vi "LINX - Blink (Simple).vi"() -> ()   [LabVIEW 2020]
uses:
  <vilib>/addons/Biomedical/Controls/Biosignal/Biosignal Spectrum/Biosignal Spectrum.xctl
  <vilib>/addons/Biomedical/Biosignal Measurements/ECG/subVIs/ECG features.ctl
  <vilib>/Analysis/3filter.llb/Filter Passband Type.ctl
  <vilib>/addons/Biomedical/Biosignal Measurements/ECG/HRV analysis/subVIs/bmt_HRV FFT Settings.ctl
  <vilib>/addons/Biomedical/Biosignal Measurements/ECG/HRV analysis/subVIs/bmt_HRV Frequency Bands.ctl
  <vilib>/addons/Biomedical/Biosignal Measurements/ECG/HRV analysis/subVIs/bmt_HRV AR Settings.ctl
  <vilib>/MakerHub/LINX/Public/Peripherals/Analog/Analog Read 1 Chan.vi
  <vilib>/MakerHub/LINX/Public/Peripherals/Analog/Analog Read N Chans.vi
  <vilib>/MakerHub/LINX/Private/Local IO/LinxAnalogRead.vi
  <vilib>/MakerHub/LINX/Public/Utilities/Check Channel.vi
  <vilib>/MakerHub/LINX/Public/Utilities/Open Serial.vi
  <vilib>/MakerHub/LINX/Private/Utilties/Generate Error.vi
  <vilib>/addons/Biomedical/Biosignal Measurements/ECG/ECG Feature Extractor (Array All).vi
  <vilib>/addons/Wavelet Analysis/application.llb/WA Detrend (Array).vi
  <vilib>/addons/Biomedical/Biosignal Measurements/ECG/HRV analysis/HRV FFT Spectrum (Array Unevenly Sampled RR).vi
  <vilib>/addons/Biomedical/Controls/Biosignal/HRV Spectrum Helper (FFT).vi
  <vilib>/addons/Biomedical/Biosignal Measurements/ECG/HRV analysis/HRV AR Spectrum (Array Unevenly Sampled RR).vi
  <vilib>/addons/Biomedical/Controls/Biosignal/HRV Spectrum Helper (AR).vi
  <vilib>/addons/Biomedical/Biosignal Measurements/ECG/HRV analysis/HRV STFT Spectrogram (Array Unevenly Sampled RR).vi
  <vilib>/addons/Time Frequency Analysis/_control.llb/TFA Configure Spectrogram Indicator (Predefined Color Table).vi
  <vilib>/MakerHub/LINX/LMH-LINX.lvlib
  <vilib>/addons/Biomedical/NI_BMTK_Measurements.lvlib
  <vilib>/ptbypt/NI_PtbyPt.lvlib
  <vilib>/Analysis/NI_AALBase.lvlib
  <vilib>/addons/Biomedical/NI_BMTK_Controls.lvlib
  <vilib>/addons/_Advanced Signal Processing/NI_AdvSigProcTFA.lvlib
  <vilib>/addons/_Advanced Signal Processing/NI_AdvSigProcWA.lvlib
panel:
  in  "Tab Control":T1(tab)
  out "NN50":i32
  out "pNN50":dbl format="%#.3g"
  out "RMSSD":dbl format="%#.3g ms"
  out "HR std":dbl format="%#.1g bpm"
  out "HR mean":dbl format="%#.1g bpm"
  out "RR std":dbl format="%#.3g s"
  out "RR mean":dbl format="%#.3g s"
  out "Count":i32
  out "RR interval histogram":T2(graph)
  out "RR triangular index":dbl format="%#_3g"
  out "TINN":dbl format="%#_3g ms"
  out "Poincare plot":cluster{"first row":dbl[], dbl[]}[](graph)
  out "SD1":dbl format="%0.2f ms"
  out "SD2":dbl format="%0.2f ms"
  out "FFT Spectrum":cluster{"f0":dbl, "df":dbl, "S(f)":dbl[]}(xcontrol)
  out "VLF Power (FFT)":dbl format="%#_2f ms^2"
  out "LF Power (FFT)":dbl format="%#_2f ms^2"
  out "HF Power (FFT)":dbl format="%#_2f ms^2"
  out "VLF [%] (FFT)":dbl format="%#_2f %"
  out "LF [%] (FFT)":dbl format="%#_2f %"
  out "HF [%] (FFT)":dbl format="%#_2f %"
  out "LF norm (FFT)":dbl format="%#_3f n.u."
  out "HF norm (FFT)":dbl format="%#_3f n.u."
  out "LF/HF (FFT)":dbl format="%#_2f"
  out "AR Spectrum":cluster{"f0":dbl, "df":dbl, "S(f)":dbl[]}(xcontrol)
  out "LF/HF (AR)":dbl format="%#_2f"
  out "HF norm (AR)":dbl format="%#_3f n.u."
  out "LF norm (AR)":dbl format="%#_3f n.u."
  out "HF [%] (AR)":dbl format="%#_2f %"
  out "LF [%] (AR)":dbl format="%#_2f %"
  out "VLF [%] (AR)":dbl format="%#_2f %"
  out "HF Power (AR)":dbl format="%#_2f ms^2"
  out "LF Power (AR)":dbl format="%#_2f ms^2"
  out "VLF Power (AR)":dbl format="%#_2f ms^2"
  out "Spectrogram":dbl[][](graph)
  out "ECG features array":T3[](array[typedef])
  out "RR interval":dbl
  out "final ECG ( without powerline noise and baseline wandering)":dbl[](graph)
  out "Statistics":T4 {"HR mean" format="%#_6f"}
  in  "Analog Input Channel":u8=13
  in  "Analyze Button":bool
  out "Loop Rate (Hz)":u32
  out "ECG without baseline wandering":dbl[](graph)
  out "original ECG":dbl[](graph)
  out "Instant Heart Rate":i32
  in  "Serial Port":refnum<visa-resource-name>
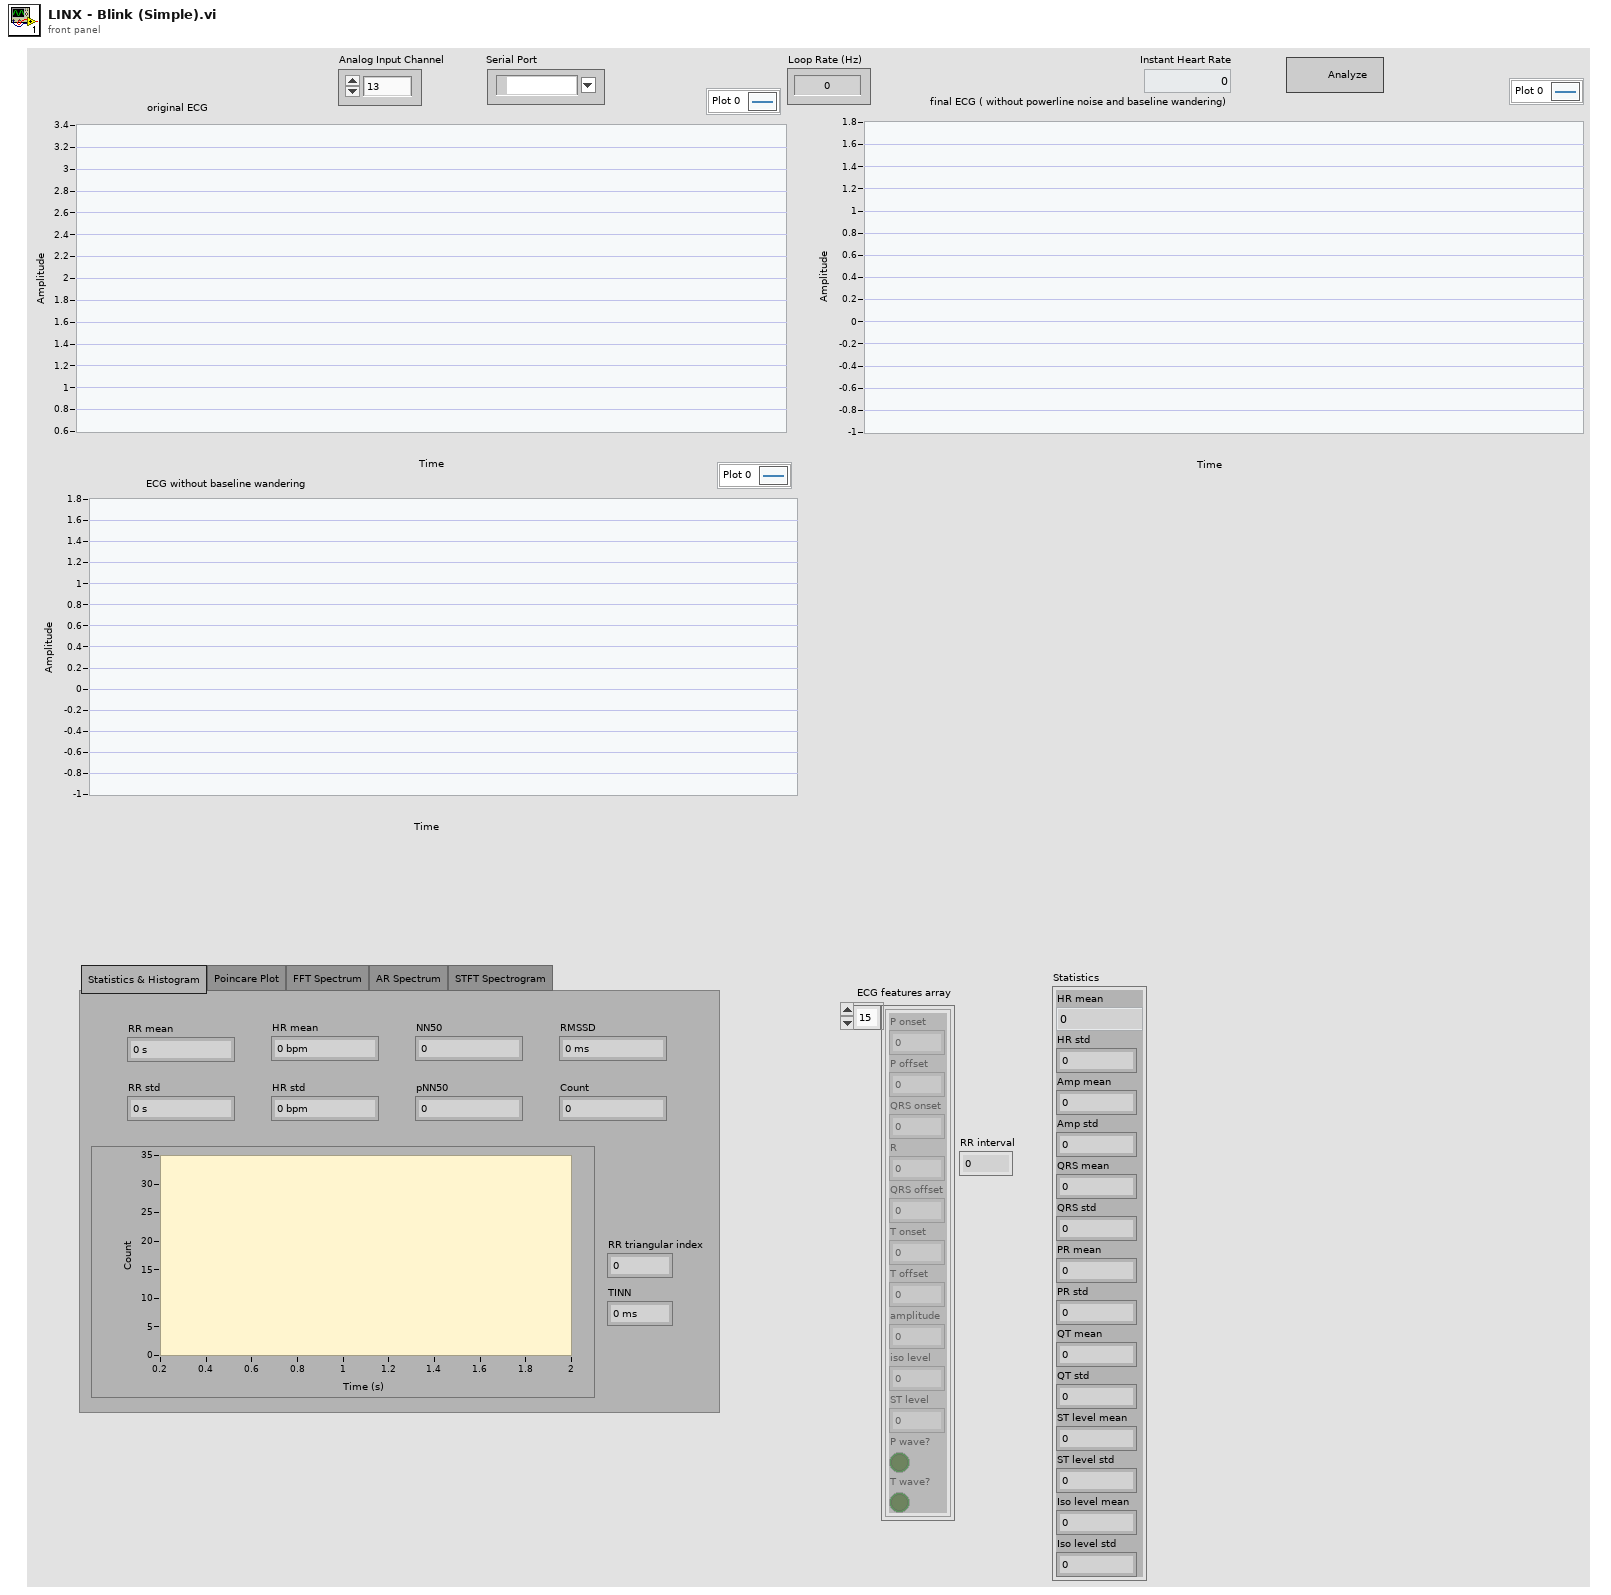
[diagram p1: front panel]
types:
  T1 = enum32{"Statistics & Histogram", "Poincare Plot", "FFT Spectrum", "AR Spectrum", "STFT Spectrogram"}
  T2 = cluster{"X Values":dbl[], "Histogram: h(x)":i32[]}
  T3 = typedef "NI_BMTK_Measurements.lvlib/ECG features.ctl" = cluster{"P onset":dbl, "P offset":dbl, "QRS onset":dbl, "R":dbl, "QRS offset":dbl, "T onset":dbl, "T offset":dbl, "amplitude":dbl, "iso level":dbl, "ST level":dbl, "P wave?":bool, "T wave?":bool}
  T4 = cluster{"HR mean":dbl, "HR std":dbl, "Amp mean":dbl, "Amp std":dbl, "QRS mean":dbl, "QRS std":dbl, "PR mean":dbl, "PR std":dbl, "QT mean":dbl, "QT std":dbl, "ST level mean":dbl, "ST level std":dbl, "Iso level mean":dbl, "Iso level std":dbl}
  T5 = typedef "NI_AALBase.lvlib/Filter Passband Type.ctl" = enum32{"Lowpass", "Highpass", "Bandpass", "Bandstop"}
  T6 = typedef "LMH-LINX.lvlib/LINX Ref.ctl" = cluster{"IO":T7, "Interface":T8, "LINX Device Config":T9}
  T7 = typedef "LMH-LINX.lvlib/Platform.ctl" = enum16{"Remote", "Local"}
  T8 = typedef "LMH-LINX.lvlib/Interface.ctl" = enum16{"Serial", "TCP"}
  T9 = typedef "LMH-LINX.lvlib/Device.lvlib/LINX Device Config.ctl" = cluster{"Interface":T8, "COM Port":refnum<visa-resource-name>, "TCP Configuration":T10, "Device Family":u8, "Device ID":u8, "Device Name":string, "TCP Ref":refnum<k5>, "Channels":T11}
  T10 = typedef "LMH-LINX.lvlib/Device.lvlib/TCP Config.ctl" = cluster{"IP Address":string, "Port":u16}
  T11 = typedef "LMH-LINX.lvlib/Channels.ctl" = cluster{"DI":u8[], "DO":u8[], "AI":u8[], "AO":u8[], "PWM":u8[], "QE":u8[], "UART":u8[], "I2C 2":u8[], "SPI":u8[], "CAN":u8[], "Servo":u8[], "AI Ref (V)":dbl, "AI Resolution (Bits)":u8, "AO Ref (V)":dbl, "AO Resolution (Bits)":u8}
  T12 = typedef "NI_BMTK_Measurements.lvlib/hrv statistics measures.ctl" = cluster{"NN50":i32, "pNN50":dbl, "RMSSD":dbl, "HR std":dbl, "HR mean":dbl, "RR std ":dbl, "RR mean":dbl}
  T13 = typedef "NI_BMTK_Measurements.lvlib/bmt_HRV FFT Settings.ctl" = cluster{"window settings":cluster{"window":u16, "length":i32, "overlap [%]":dbl}, "frequency bands":T14, "dB on? (F)":bool, "frequency bins":i32}
  T14 = typedef "NI_BMTK_Measurements.lvlib/bmt_HRV Frequency Bands.ctl" = cluster{"VLF high":dbl, "VLF low":dbl, "LF high":dbl, "LF low":dbl, "HF high":dbl, "HF low":dbl}
  T15 = typedef "NI_BMTK_Measurements.lvlib/bmt_Spectrum Meatures.ctl" = cluster{"VLF peak frequency":dbl, "VLF peak amplitude ":dbl, "LF peak frequency ":dbl, "LF peak amplitude ":dbl, "HF peak frequency":dbl, "HF peak amplitude":dbl, "VLF power":dbl, "LF power":dbl, "HF power":dbl, "LF norm":dbl, "HF norm":dbl, "LF/HF":dbl, "VLF [%]":dbl, "LF [%]":dbl, "HF [%]":dbl}
  T16 = typedef "NI_BMTK_Measurements.lvlib/bmt_HRV AR Settings.ctl" = cluster{"frequency bands":T14, "dB on? (F)":bool, "method":u16, "order":i32, "frequency bins":i32}
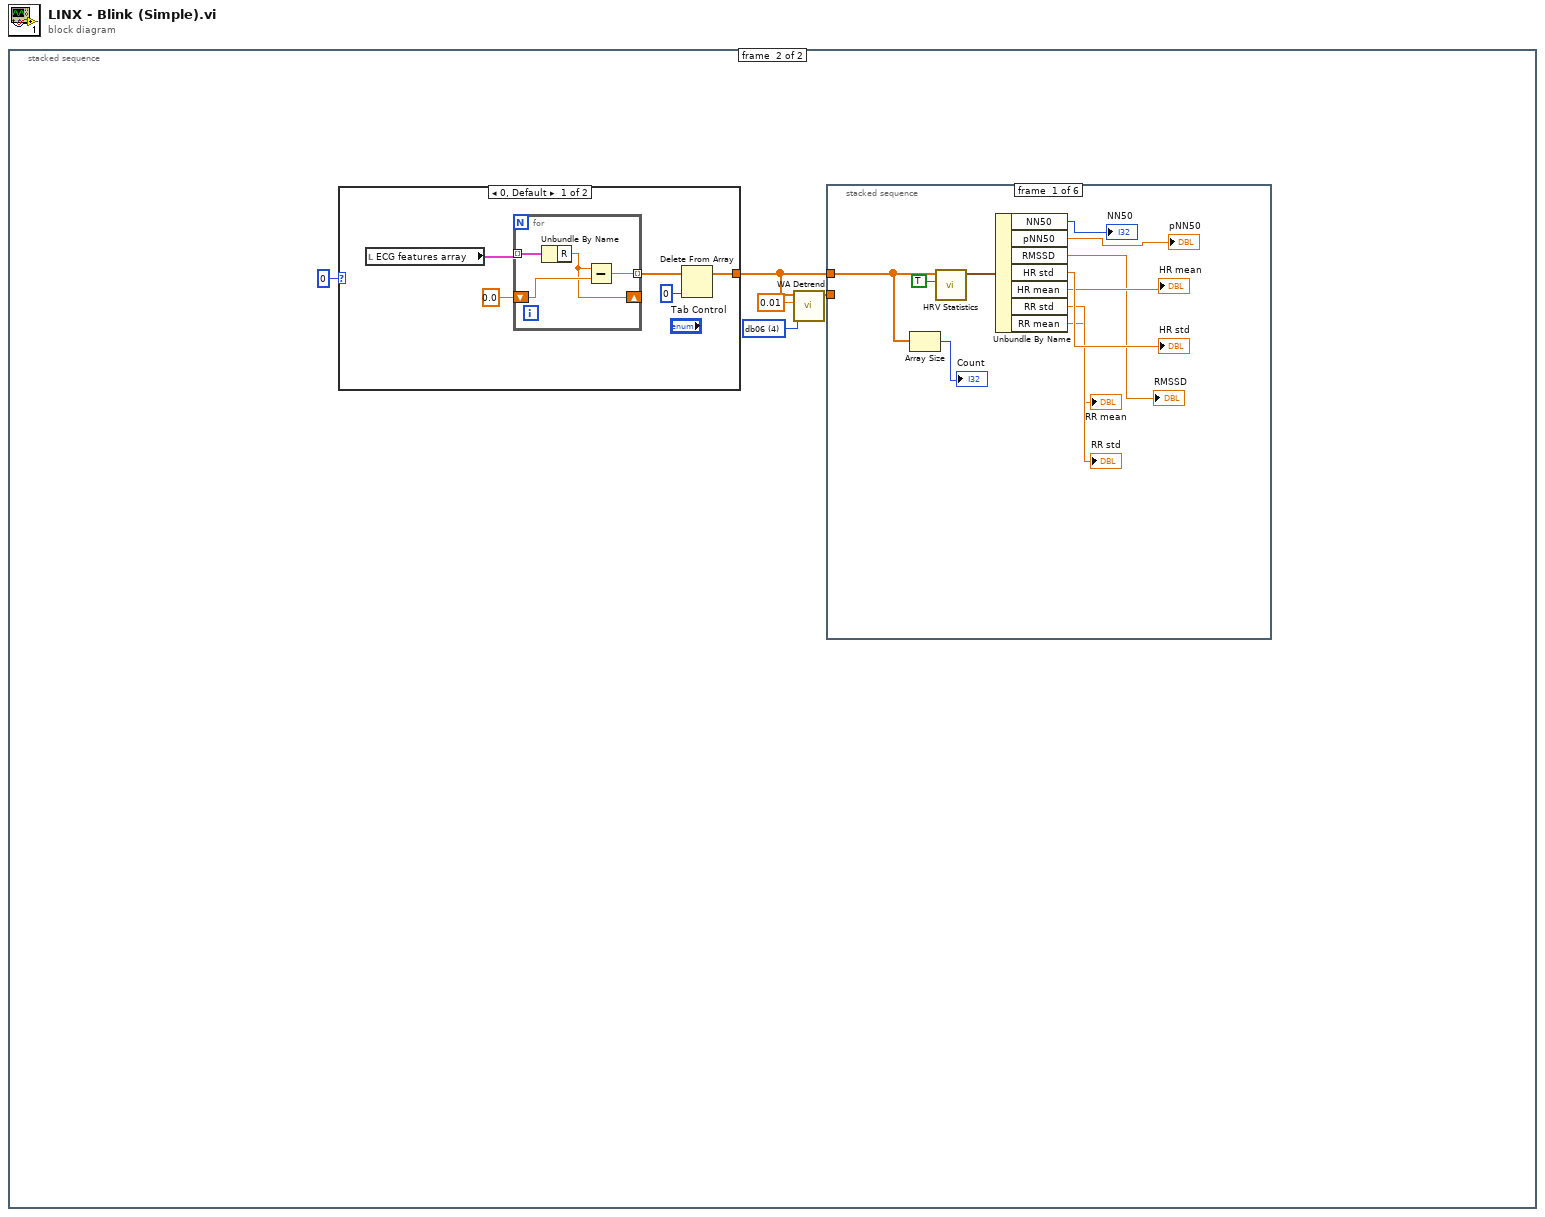
[diagram p0: block diagram]
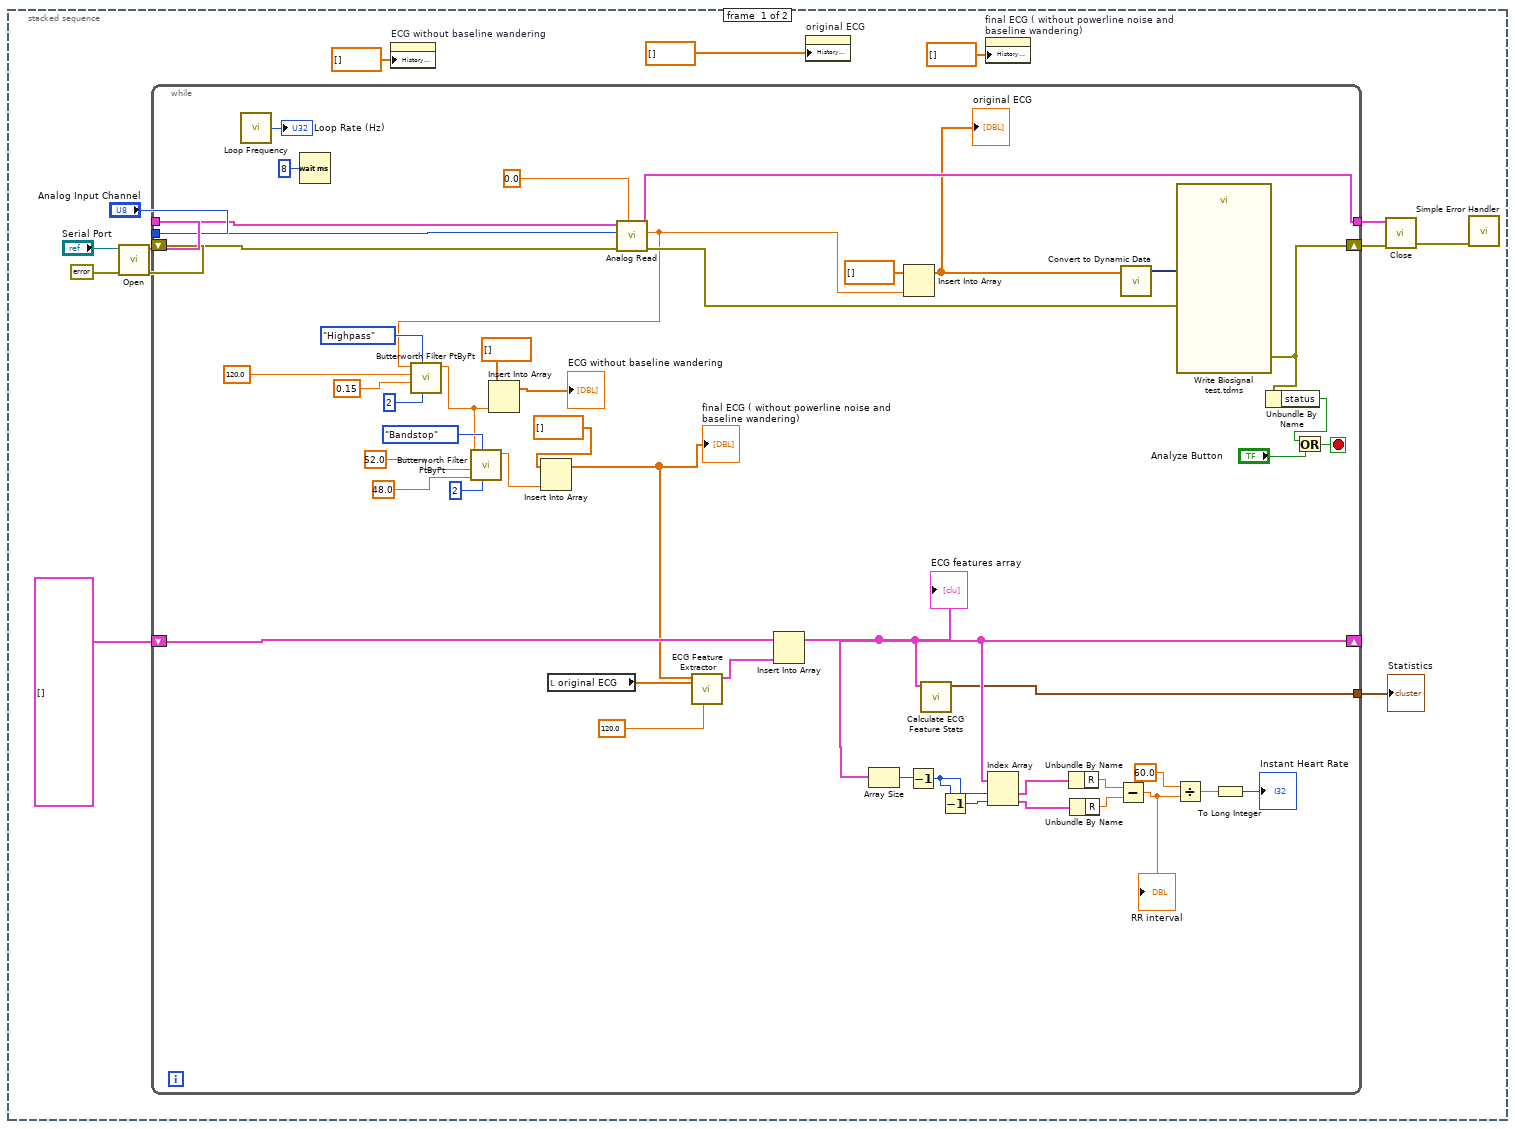
[diagram p2: hidden frame]
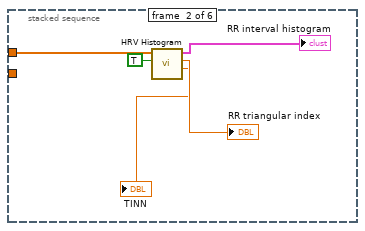
[diagram p3: hidden frame]
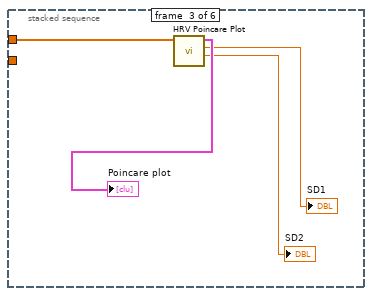
[diagram p4: hidden frame]
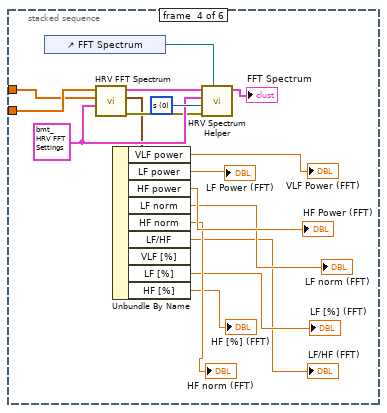
[diagram p5: hidden frame]
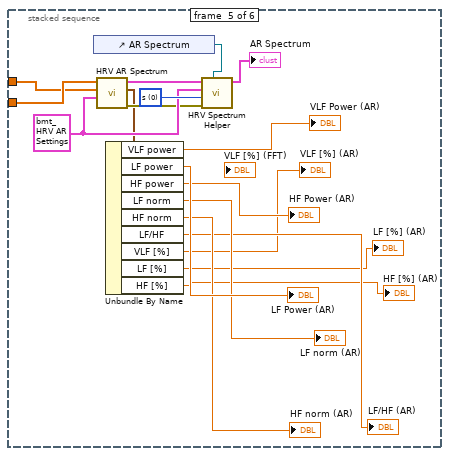
[diagram p6: hidden frame]
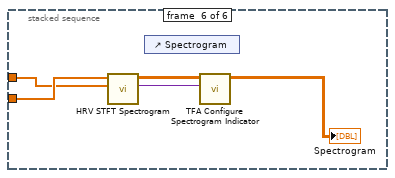
[diagram p7: hidden frame]
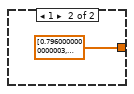
[diagram p8: hidden frame]
diagram:
  n1 = stacked-sequence {
    frame #0 {
      n2 = call-poly <vilib>:"Open.vi"("Error In"=errorcluster {"status"=FALSE, "code"=0, "source"=""}, "Serial Port"="Serial Port") -> ("Error Out"=w12:errorcluster, "LINX Resource"=w13:T6)  [unwired: 7 in, 1 out]
      n3 = while {
        tunnel: w13 -> [w58]
        tunnel: [w57] -> w11
        shift-right: [w35] -> w10
        shift-left: w12 -> [w47]
        tunnel: "Analog Input Channel" -> [w55]
        shift-right: [w33] -> _
        shift-left: T3[] [] ("array") -> [w49]
        tunnel: [w16] -> w4
        stop <- w60 stop-if-true
        n4 = call <vilib>:"Loop Frequency.vi"() -> ("Loop Rate (Hz)"=→"Loop Rate (Hz)":u32)
        n5 = Wait (ms)(milliseconds to wait=u32 8) -> ()  [unwired: 1 out]
        n6 = local read "original ECG"() -> (w24:dbl[])
        n7 = call-poly <vilib>:"Analog Read.vi"("Analog Ref Override (V)"=0.0, "Error In"=w47, "Analog Channel"=w55, "LINX Resource"=w58) -> ("Error Out"=w34:errorcluster, "Voltage"=w27:dbl, "LINX Resource"=w57:T6)  [unwired: 4 in, 1 out]
        n8 = call <vilib>:"Butterworth Filter PtByPt.vi"("order"=2, "filter type"=Filter_Passband_Type."Highpass", "high cutoff freq: fh"=0.15, "sampling freq: fs"=120.0, "x"=w27) -> ("Filtered x"=w22:dbl)  [unwired: 4 in, 1 out]
        n9 = call <vilib>:"Butterworth Filter PtByPt.vi"("order"=2, "filter type"=Filter_Passband_Type."Bandstop", "low cutoff freq: fl"=48.0, "high cutoff freq: fh"=52.0, "x"=w22) -> ("Filtered x"=w18:dbl)  [unwired: 4 in, 1 out]
        n10 = Insert Into Array(array=dbl[] [], new element=w22) -> (→"ECG without baseline wandering":dbl[])  [unwired: 1 in]
        n11 = Insert Into Array(array=dbl[] [], new element=w18) -> (w15:dbl[])  [unwired: 1 in]
        "final ECG ( without powerline noise and baseline wandering)" <- w15
        n12 = call-poly <vilib>:"ECG Feature Extractor.vi"("sampling rate"=120.0, "raw ECG"=w24, "ECG"=w15) -> ("ECG features"=w50:T3[])  [unwired: 7 in, 1 out]
        n13 = Insert Into Array(array=w49, new element=w50) -> (w33:T3[])  [unwired: 1 in]
        "ECG features array" <- w33
        n14 = Array Size(array=w33) -> (size(s)=w46:i32)
        n15 = Insert Into Array(array=dbl[] [], new element=w27) -> (w32:dbl[])  [unwired: 1 in]
        "original ECG" <- w32
        n16 = Decrement(x=w46) -> (x-1=w45:i32)
        n17 = call "Calculate ECG Feature Stats.vi"("ECG Features"=w33) -> ("Statistics"=w16:T4)  [unwired: 10 in]
        n18 = Decrement(x=w45) -> (x-1=w44:i32)
        n19 = Index Array(array=w33, index #1=w45, index #2=w44) -> (element #1=w43:T3, element #2=w42:T3)
        n20 = Unbundle By Name(w43) -> ("R"=w41:dbl)
        n21 = Unbundle By Name(w42) -> ("R"=w40:dbl)
        n22 = Subtract(x=w41, y=w40) -> (x-y=w14:dbl)
        "RR interval" <- w14
        n23 = call "Convert to Dynamic Data"("Array"=w32) -> ("Dynamic Data Type"=w51:dynamicdata)  [unwired: 3 in]
        n24 = Divide(x=60.0, y=w14) -> (x/y=w39:dbl)
        n25 = call "Write Biosignal\ntest.tdms"("error in (no error)"=w34, "biosignals"=w51) -> ("error out"=w35:errorcluster)  [unwired: 9 in]
        n26 = To Long Integer(number=w39) -> (32bit integer=→"Instant Heart Rate":i32)
        n27 = Unbundle By Name(w35) -> ("status"=w36:bool)
        n28 = Or(x=w36, y="Analyze Button") -> (x .or. y?=w60:bool)
      }
      "Statistics" <- w4
      n29 = property on="ECG without baseline wandering" class="WFChart (strict)"("History Data"=dbl[] []) -> ()  [unwired: 2 in, 2 out]
      n30 = property on="original ECG" class="WFChart (strict)"("History Data"=dbl[] []) -> ()  [unwired: 2 in, 2 out]
      n31 = property on="final ECG ( without powerline noise and baseline wandering)" class="WFChart (strict)"("History Data"=dbl[] []) -> ()  [unwired: 2 in, 2 out]
      n32 = call <vilib>:"Close.vi"("Error In"=w10, "LINX Resource"=w11) -> ("Error Out"=w8:errorcluster)  [unwired: 9 in]
      n33 = call <vilib>:"Simple Error Handler.vi"("error in (no error)"=w8) -> ()  [unwired: 4 in, 5 out]
    }
    frame #1 {
      w65 = u16 4 items=["db02"=0, "db03"=1, "db04"=2, "db05"=3, "db06"=4, "db07"=5, "db08"=6, "db09"=7, "db10"=8, "db11"=9, "db12"=10, "db13"=11, "db14"=12, "Haar"=13, "bior1_3"=14, "bior1_5"=15, "bior2_2"=16, "bior2_4"=17, "bior2_6"=18, "bior2_8"=19, "bior3_1"=20, "bior3_3"=21, "bior3_5"=22, "bior3_7"=23, "bior3_9"=24, "bior4_4 (FBI)"=25, "bior5_5"=38, "bior6_8"=39, "coif1"=26, "coif2"=27, "coif3"=28, "coif4"=29, "coif5"=30, "sym2"=31, "sym3"=32, "sym4"=33, "sym5"=34, "sym6"=35, "sym7"=36, "sym8"=37] ("wavelet")
      n34 = case shown="0, Default" u16 0 ("RR Interval Source") {
        tunnel: [w127 dbl[] [0.7960000000000003, 0.8160000000000007, 0.8379999999999992, 0.8460000000000001, 0.8260000000000005, 0.8279999999999994, 0.8059999999999992, 0.75, 0.7080000000000002, 0.7140000000000004, 0.7279999999999998, 0.6899999999999995, 0.7200000000000024, 0.7620000000000005, 0.8079999999999998, 0.8019999999999996, 0.8339999999999996, 0.8439999999999976, 0.8399999999999999, 0.8300000000000018, 0.8240000000000016, 0.8299999999999983, 0.8320000000000007, 0.8320000000000007, 0.8239999999999981, 0.8360000000000021, 0.847999999999999, 0.8580000000000005, 0.8359999999999985, 0.8260000000000005, 0.8619999999999983, 0.8540000000000028, 0.8500000000000014, 0.8499999999999943, 0.8640000000000043, 0.8659999999999997, 0.8680000000000021, 0.8239999999999981, 0.8200000000000003, 0.7520000000000024, 0.75, 0.7239999999999966, 0.7839999999999989, 0.8340000000000032, 0.8419999999999987, 0.8260000000000005, 0.7980000000000018, 0.8239999999999981, 0.8159999999999954, 0.7860000000000014, 0.7760000000000034, 0.7899999999999991, 0.8100000000000023, 0.8099999999999952, 0.8079999999999998, 0.8000000000000043, 0.7959999999999994, 0.7680000000000007, 0.7860000000000014, 0.7939999999999969, 0.804000000000002, 0.7999999999999972, 0.8100000000000023, 0.8320000000000007, 0.5899999999999963, 1.0500000000000043, 0.8639999999999972, 0.8539999999999992, 0.8599999999999994, 0.8599999999999994, 0.8380000000000081, 0.8539999999999992, 0.7920000000000016, 0.8059999999999974, 0.7879999999999967, 0.7800000000000011, 0.8019999999999925, 0.7960000000000065, 0.7420000000000044, 0.7740000000000009, 0.8019999999999925, 0.7900000000000063, 0.7920000000000016, 0.8099999999999881, 0.8080000000000069, 0.7819999999999965, 0.7960000000000065, 0.8100000000000023, 0.7959999999999923, 0.7259999999999991, 0.75, 0.7459999999999951, 0.7260000000000133, 0.7479999999999905, 0.7280000000000086, 0.7620000000000005, 0.7959999999999923, 0.8340000000000032, 0.8259999999999934, 0.8359999999999985, 0.8540000000000134, 0.8619999999999948, 0.8359999999999985, 0.828000000000003, 0.8460000000000036, 0.8239999999999981, 0.7959999999999923, 0.8200000000000074, 0.804000000000002, 0.7879999999999967, 0.7259999999999991, 0.7459999999999951, 0.7660000000000053, 0.7800000000000011, 0.8019999999999925, 0.7700000000000102, 0.7680000000000007, 0.789999999999992, 0.7879999999999967, 0.7700000000000102, 0.7979999999999876, 0.8080000000000069, 0.8100000000000023, 0.8019999999999925, 0.7319999999999993, 0.7400000000000091, 0.7519999999999953, 0.7420000000000044, 0.7339999999999947, 0.7379999999999995, 0.7379999999999995, 0.7180000000000035, 0.7120000000000033, 0.7379999999999995, 0.7639999999999958, 0.7439999999999998, 0.7960000000000065, 0.8019999999999925, 0.7920000000000016, 0.8179999999999978, 0.8260000000000076, 0.8119999999999976, 0.8199999999999932, 0.8340000000000032, 0.8419999999999987, 0.7860000000000014, 0.8080000000000069, 0.8019999999999925, 0.8100000000000023, 0.8059999999999974, 0.7999999999999972, 0.7280000000000086, 0.7119999999999891, 0.7379999999999995, 0.7980000000000018, 0.8259999999999934, 0.8200000000000216, 0.8400000000000034, 0.8439999999999941, 0.8239999999999839, 0.75, 0.6980000000000075, 0.7139999999999986, 0.75, 0.8060000000000116, 0.8400000000000034, 0.8559999999999945, 0.8640000000000043, 0.8639999999999759, 0.8340000000000032, 0.8500000000000227, 0.8079999999999927, 0.828000000000003, 0.8340000000000032, 0.8179999999999836, 0.8199999999999932, 0.8000000000000114, 0.8199999999999932, 0.7920000000000016, 0.7960000000000207, 0.8179999999999836, 0.8360000000000127, 0.804000000000002, 0.8019999999999925, 0.7959999999999923, 0.7680000000000007, 0.7340000000000089, 0.7179999999999893, 0.7060000000000173, 0.7199999999999989, 0.7519999999999811, 0.7900000000000205, 0.8219999999999743, 0.842000000000013, 0.8220000000000027, 0.8079999999999927, 0.8379999999999939, 0.832000000000022, 0.8219999999999743, 0.7800000000000011, 0.7720000000000198, 0.7419999999999902, 0.7079999999999984, 0.7220000000000084, 0.7460000000000093, 0.7839999999999918, 0.8439999999999941, 0.8100000000000023, 0.7800000000000011, 0.7959999999999923, 0.8079999999999927, 0.8260000000000218, 0.8220000000000027, 0.8239999999999839, 0.7839999999999918, 0.7800000000000011, 0.7860000000000014, 0.8000000000000114, 0.8060000000000116, 0.8099999999999739, 0.8120000000000118, 0.8079999999999927, 0.7860000000000014, 0.7840000000000202, 0.8059999999999832, 0.8220000000000027, 0.7779999999999916, 0.7880000000000109, 0.8160000000000025, 0.8319999999999936, 0.8199999999999932, 0.7940000000000111, 0.7299999999999898, 0.7280000000000086, 0.7319999999999993, 0.7319999999999993, 0.7239999999999895, 0.7040000000000077, 0.7299999999999898, 0.7560000000000002, 0.7820000000000107, 0.7880000000000109, 0.7579999999999814, 0.7520000000000095, 0.7299999999999898, 0.7060000000000173, 0.7279999999999802, 0.7420000000000186, 0.7319999999999993, 0.7460000000000093, 0.7279999999999802, 0.7439999999999998, 0.7700000000000102, 0.789999999999992, 0.813999999999993, 0.8080000000000211, 0.7939999999999827, 0.8260000000000218, 0.799999999999983, 0.8000000000000114, 0.7620000000000005, 0.7620000000000005, 0.7719999999999914, 0.7179999999999893, 0.7340000000000089, 0.7280000000000086, 0.7379999999999995, 0.7259999999999991, 0.7059999999999889, 0.724000000000018, 0.7319999999999993, 0.7479999999999905, 0.7400000000000091, 0.7279999999999802, 0.724000000000018, 0.72199999999998, 0.710000000000008, 0.7340000000000089, 0.7620000000000005, 0.7860000000000014, 0.7779999999999916, 0.789999999999992, 0.8080000000000211, 0.8179999999999836, 0.7959999999999923, 0.8120000000000118, 0.8160000000000025, 0.813999999999993, 0.8019999999999925, 0.8200000000000216, 0.8239999999999839, 0.8100000000000023, 0.8120000000000118, 0.8259999999999934, 0.8220000000000027, 0.804000000000002, 0.7819999999999823, 0.7900000000000205, 0.8239999999999839, 0.8000000000000114, 0.7939999999999827, 0.8100000000000023, 0.8160000000000025, 0.818000000000012, 0.7920000000000016, 0.804000000000002, 0.799999999999983, 0.7860000000000014, 0.7900000000000205, 0.7839999999999918, 0.799999999999983, 0.8200000000000216, 0.799999999999983, 0.8100000000000023, 0.8460000000000036, 0.8319999999999936, 0.79200000000003, 0.7559999999999718, 0.7560000000000286, 0.7620000000000005, 0.7319999999999709, 0.7420000000000186, 0.7459999999999809, 0.7459999999999809, 0.6920000000000073, 0.6860000000000355, 0.6979999999999791, 0.7160000000000082, 0.7199999999999704, 0.7000000000000455, 0.69399999999996, 0.6899999999999977, 0.6820000000000164, 0.6999999999999886, 0.7520000000000095, 0.7459999999999809, 0.7560000000000286, 0.7679999999999723, 0.7960000000000491, 0.7539999999999623, 0.7760000000000105, 0.8059999999999832, 0.7900000000000205, 0.7420000000000186, 0.76400000000001, 0.7980000000000018, 0.8159999999999741, 0.77800000000002, 0.7999999999999545, 0.80600000000004, 0.8100000000000023, 0.7799999999999727, 0.73599999999999, 0.7460000000000377, 0.7639999999999532, 0.7960000000000491, 0.7639999999999532, 0.7100000000000364, 0.7119999999999891, 0.7339999999999804, 0.7700000000000387, 0.8039999999999736, 0.8380000000000223, 0.8319999999999936, 0.8319999999999936, 0.8380000000000223, 0.8340000000000032, 0.8159999999999741, 0.8199999999999932, 0.8160000000000309, 0.7959999999999923, 0.8100000000000023, 0.8019999999999641, 0.7880000000000109, 0.7939999999999827, 0.7420000000000186, 0.7620000000000005, 0.7740000000000009, 0.7880000000000109, 0.7760000000000105, 0.7819999999999823, 0.7420000000000186, 0.7559999999999718] ("Array")] -> w63
        frame 0, Default {
          n35 = local read "ECG features array"() -> (w126:T3[])
          n36 = for {
            tunnel: w126 -> [w134] mode=indexing
            shift-right: [w132] -> _
            shift-left: 0.0 -> [w133]
            tunnel: [w131] -> w129 mode=indexing
            n37 = Unbundle By Name(w134) -> ("R"=w132:dbl)
            n38 = Subtract(x=w132, y=w133) -> (x-y=w131:dbl)
          }
          n39 = Delete From Array(array=w129, index=0) -> (array with subset deleted=w127:dbl[])  [unwired: 1 in, 1 out]
        }
        frame 1 {
        }
      }
      n40 = call-poly <vilib>:"WA Detrend.vi"("wavelet"=w65, "threshold frequency"=0.01, "signal"=w63) -> ("detrended signal"=w62:dbl[])  [unwired: 6 in, 2 out]
      n41 = stacked-sequence {
        tunnel: w63 -> [w74 w80 w85 w97 w115 w124]
        tunnel: w62 -> [_ _ _ w98 w116 w125]
        frame #0 {
          n42 = Array Size(array=w74) -> (size(s)=→"Count":i32)
          n43 = call <vilib>:"HRV Statistics.vi"("detrend? (F)"=TRUE, "raw RR"=w74) -> ("statistics measurements"=w76:T12)  [unwired: 8 in, 1 out]
          n44 = Unbundle By Name(w76) -> ("NN50"=→"NN50":i32, "pNN50"=→"pNN50":dbl, "RMSSD"=→"RMSSD":dbl, "HR std"=→"HR std":dbl, "HR mean"=→"HR mean":dbl, "RR std"=→"RR std":dbl, "RR mean"=→"RR mean":dbl)
        }
        frame #1 {
          n45 = call <vilib>:"HRV Histogram.vi"("detrend? (F)"=TRUE, "raw RR"=w80) -> ("TINN"=→"TINN":dbl, "RR triangular index"=→"RR triangular index":dbl, "RR interval histogram"=→"RR interval histogram":T2)  [unwired: 4 in, 3 out]
        }
        frame #2 {
          n46 = call <vilib>:"HRV Poincare Plot.vi"("raw RR"=w85) -> ("SD2"=→"SD2":dbl, "SD1"=→"SD1":dbl, "Poincare plot"=→"Poincare plot":cluster{"first row":dbl[], dbl[]}[])  [unwired: 5 in, 3 out]
        }
        frame #3 {
          w100 = T13 {"window settings"={"window"=1, "length"=1024, "overlap [%]"=50.0}, "frequency bands"={"VLF high"=0.04, "VLF low"=0.0, "LF high"=0.15, "LF low"=0.04, "HF high"=0.4, "HF low"=0.15}, "dB on? (F)"=FALSE, "frequency bins"=1024} ("FFT setttings")
          w102 = u16 0 items=["s", "ms"] ("RR unit")
          n47 = control-ref of="FFT Spectrum"() -> (w86:refnum<vi>)
          n48 = call-poly <vilib>:"HRV FFT Spectrum.vi"("FFT settings"=w100, "raw RR"=w97, "RR"=w98) -> ("error out"=w99:errorcluster, "FFT measurements"=w96:T15, "FFT spectrum"=w101:cluster{"f0":dbl, "df":dbl, "S(f)":dbl[]})  [unwired: 6 in]
          n49 = Unbundle By Name(w96) -> ("VLF power"=→"VLF Power (FFT)":dbl, "LF power"=→"LF Power (FFT)":dbl, "HF power"=→"HF Power (FFT)":dbl, "LF norm"=→"LF norm (FFT)":dbl, "HF norm"=→"HF norm (FFT)":dbl, "LF/HF"=→"LF/HF (FFT)":dbl, "LF [%]"=→"LF [%] (FFT)":dbl, "HF [%]"=→"HF [%] (FFT)":dbl)  [unwired: 1 out]
          n50 = call-poly <vilib>:"HRV Spectrum Helper.vi"("HRV spectrum"=w86, "error in (no error)"=w99, "RR unit"=w102, "FFT settings"=w100, "spectrum in"=w101) -> ("spectrum out"=→"FFT Spectrum":cluster{"f0":dbl, "df":dbl, "S(f)":dbl[]})  [unwired: 5 in, 1 out]
        }
        frame #4 {
          w120 = u16 0 items=["s", "ms"] ("RR unit")
          w118 = T16 {"frequency bands"={"VLF high"=0.04, "VLF low"=0.0, "LF high"=0.15, "LF low"=0.04, "HF high"=0.4, "HF low"=0.15}, "dB on? (F)"=FALSE, "method"=0, "order"=16, "frequency bins"=1024} ("AR settings")
          n51 = control-ref of="AR Spectrum"() -> (w112:refnum<vi>)
          n52 = call-poly <vilib>:"HRV AR Spectrum.vi"("AR settings"=w118, "raw RR"=w115, "RR"=w116) -> ("error out"=w117:errorcluster, "AR measurements"=w114:T15, "AR spectrum"=w119:cluster{"f0":dbl, "df":dbl, "S(f)":dbl[]})  [unwired: 6 in]
          n53 = Unbundle By Name(w114) -> ("VLF power"=→"VLF Power (AR)":dbl, "LF power"=→"LF Power (AR)":dbl, "HF power"=→"HF Power (AR)":dbl, "LF norm"=→"LF norm (AR)":dbl, "HF norm"=→"HF norm (AR)":dbl, "LF/HF"=→"LF/HF (AR)":dbl, "VLF [%]"=→"VLF [%] (AR)":dbl, "LF [%]"=→"LF [%] (AR)":dbl, "HF [%]"=→"HF [%] (AR)":dbl)
          n54 = call-poly <vilib>:"HRV Spectrum Helper.vi"("HRV spectrum"=w112, "error in (no error)"=w117, "RR unit"=w120, "AR settings"=w118, "spectrum in"=w119) -> ("spectrum out"=→"AR Spectrum":cluster{"f0":dbl, "df":dbl, "S(f)":dbl[]})  [unwired: 5 in, 1 out]
        }
        frame #5 {
          n55 = call-poly <vilib>:"HRV STFT Spectrogram.vi"("raw RR"=w124, "RR"=w125) -> ("scale info"=w122:variant, "spectrogram"=w123:dbl[][])  [unwired: 7 in, 1 out]
          n56 = control-ref of="Spectrogram"() -> ()  [unwired: 1 out]
          n57 = call-poly <vilib>:"TFA Configure Spectrogram Indicator.vi"("scale info"=w122, "spectrogram"=w123) -> ("TF spectrogram indicator"=→"Spectrogram":dbl[][])  [unwired: 5 in, 4 out]
        }
      }
    }
  }
